vi "Clear.vi"(8 "error in (no error)":errorcluster, 11 "Error Code":i32) -> (0 "error out":errorcluster)   [LabVIEW 2026, in "TALOS.lvlib" / "Classes.lvlib" / "Error Filter.lvclass"]
doc: "Use this VI to add an error to be skipped in the future. If repetitions and time are both left to zero, the error will be permanently skipped: otherwise the error will be skipped until at least one of the two conditions will be met."
uses:
  Error Filter.lvclass
  Ancestor/Ancestor/Ancestor.lvclass/Ancestor.ctl
  Support VIs/Generate Error.vi
  FGV/Error Memory/Get Error Description.vi
  Support VIs/Get PC name.vi
  Ancestor/Ancestor/Read ID.vi
  Support VIs/Get Class Name.vi
  <vilib>/Utility/error.llb/Clear Errors.vi
  FGV/Error Memory/Error Memory Core.vi
  <vilib>/AdvancedString/Delimited String to 1D String Array.vi
  <vilib>/AdvancedString/Delimited String to 1D String Array (string).vi
  Support VIs/Circus Root Path.vi
  FGV/Error Memory/Error Crt Lvl checker.vi
  FGV/Error Memory/Error Memory Core.vi/40c8088d-b597-4017-91af-faa98e00292e.vi
  FGV/Error Memory/Error Memory Core.vi/d4a3ab98-063c-4e44-b43d-fbdcfe6c2be2.vi
  Support VIs/Global Memory.vi
  <vilib>/Utility/LVClass/Get LV Class Name.vi
  Support VIs/Is in Packed Library.vi
  Support VIs/TALOS Root path.vi
  Support VIs/Read CSV worksheet.vi
  Support VIs/Global Constants.vi
  <vilib>/Utility/error.llb/General Error Handler.vi
  Support VIs/Error Log.vi
  Ancestor/Ancestor/Ancestor.lvclass
  <vilib>/Comparison/Equal/Equal Functor/Equal Functor.lvclass
  TALOS.lvlib
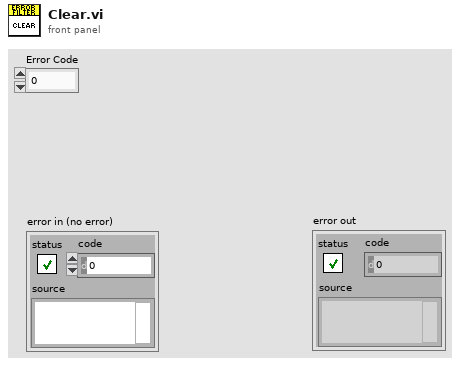
[diagram p1: front panel]
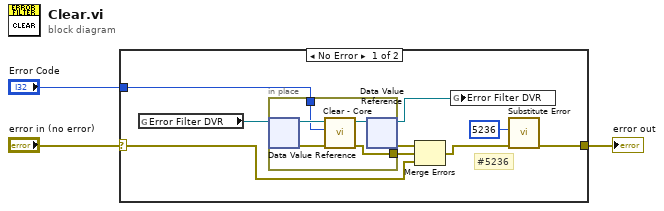
[diagram p0: block diagram]
diagram:
  n1 = case shown="No Error" "error in (no error)" {
    selector: "error in (no error)" -> [w12 w18]
    tunnel: [w10 w18] -> w1
    tunnel: "Error Code" -> [w7 _]
    frame No Error {
      # "#5236"
      n2 = global read "Global Memory.vi" "Error Filter DVR"() -> (w9:refnum<data-value>)
      n3 = in-place {
        in-place-border: w7 -> [w13]
        in-place-border: [w14] -> w6
        n4 = in-place-dvr #1(w9) -> (w17:refnum<class "Error Filter.lvclass">, w15:errorcluster)
        n5 = call "Clear - Core.vi"("error in (no error)"=w15, "Error Code"=w13, "Error Filter in"=w17) -> ("error out"=w14:errorcluster, "Error Filter out"=w16:refnum<class "Error Filter.lvclass">)  [unwired: 7 in]
        n6 = in-place-dvr #1(w16) -> (w5:refnum<data-value>, w8:errorcluster)
      }
      n7 = Merge Errors(w8, w6, w12) -> (w11:errorcluster)
      n8 = global write "Global Memory.vi" "Error Filter DVR"(w5) -> ()
      n9 = call "Substitute Error.vi"("error in (no error)"=w11, "Error Code"=5236) -> ("error out"=w10:errorcluster)  [unwired: 9 in]
    }
    frame Error {
    }
  }
  "error out" <- w1
